vi "ZMC Read Message.vi"(7 "puiread":u32, 8 "error in (no error)":errorcluster caption="错误输入（无错误）", 9 "uimax":u32, 10 "pbuff":string, 11 "handle":u32) -> (0 "error out":errorcluster caption="错误输出", 1 "function return":i32, 2 "pbuff out":string, 3 "handle out":u32, 5 "puiread out":u32)   [LabVIEW 2015, in "zauxdll.lvlib"]
doc: "int32 __stdcall ZMC_ReadMessage(ZMC_HANDLE handle, char * pbuff, uint32 uimax, uint32 *puiread);"
uses:
  zauxdll.lvlib
  zmotion.dll
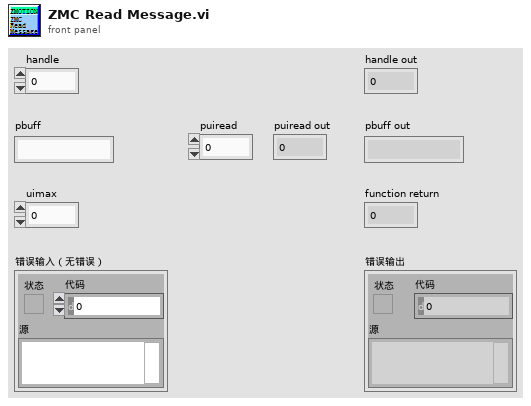
[diagram p1: front panel]
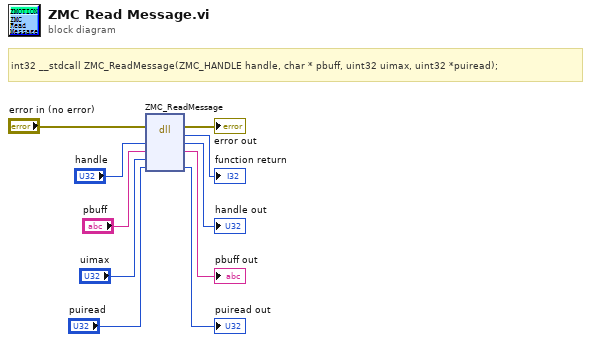
[diagram p0: block diagram]
diagram:
  # "int32 __stdcall ZMC_ReadMessage(ZMC_HANDLE handle, char * pbuff, uint32 uimax, uint32 *puiread);"
  n1 = dll-call lib="C:/Users/VIC/Desktop/GOGORO_SA/system/LLB/zmotion/zaux/zmotion.*" fn="ZMC_ReadMessage"(error in="error in (no error)", "handle"="handle", "pbuff"="pbuff", "uimax"="uimax", "puiread"="puiread") -> (error out=→"error out":errorcluster, →"function return":i32, "handle"=→"handle out":u32, "pbuff"=→"pbuff out":string, "puiread"=→"puiread out":u32)  [unwired: 3 in, 1 out]
